vi "Update Controls in UI.vi"(4 "9216 Config":T3 {"RTD_Type" items=["TCR3851"=1, "TCR3750"=2, "TCR3916"=3, "TCR3920"=4, "TCR3911"=5, "TCR3928"=6, "Custom"=0]; "Degree Range" items=["Raw Ohms", "Degrees Kelvin", "Degrees Celsius", "Degrees Fahrenheit", "Degrees Rankine"]; "Conversion Time" items=["200 ms", "2.5 ms"]}, 6 "Values":i32[](array[numeric])=[0], 8 "RTD Type":u8, 9 "Units":u8, 10 "RTD coefficients":T1, 11 "RTD types and units controls":cluster{"controls":T2, "typedefs":T2}) -> ()   [LabVIEW 2020, in "Modules.lvlib" / "9216.lvclass"]
uses:
  9216.lvclass
  RTD Rings for Type and Units.ctl
  RTD Coefficients.ctl
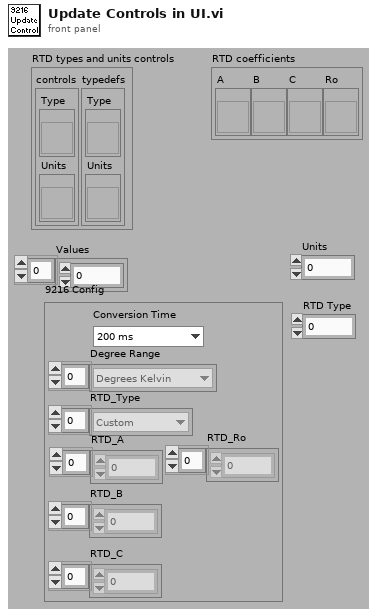
[diagram p1: front panel]
types:
  T1 = typedef "Modules.lvlib/9216.lvclass/RTD Coefficients.ctl" = cluster{"A":refnum<vi>, "B":refnum<vi>, "C":refnum<vi>, "Ro":refnum<vi>}
  T2 = typedef "Modules.lvlib/9216.lvclass/RTD Rings for Type and Units.ctl" = cluster{"Type":refnum<vi>, "Units":refnum<vi>}
  T3 = cluster{"Conversion Time":u16, "Degree Range":u8[], "RTD_Type":u8[], "RTD_A":dbl[], "RTD_B":dbl[], "RTD_C":dbl[], "RTD_Ro":dbl[]}
  T4 = typedef "LVStringsAndValuesArrayTypeDef_U8.ctl" = cluster{"String":string, "Value":u8}[]
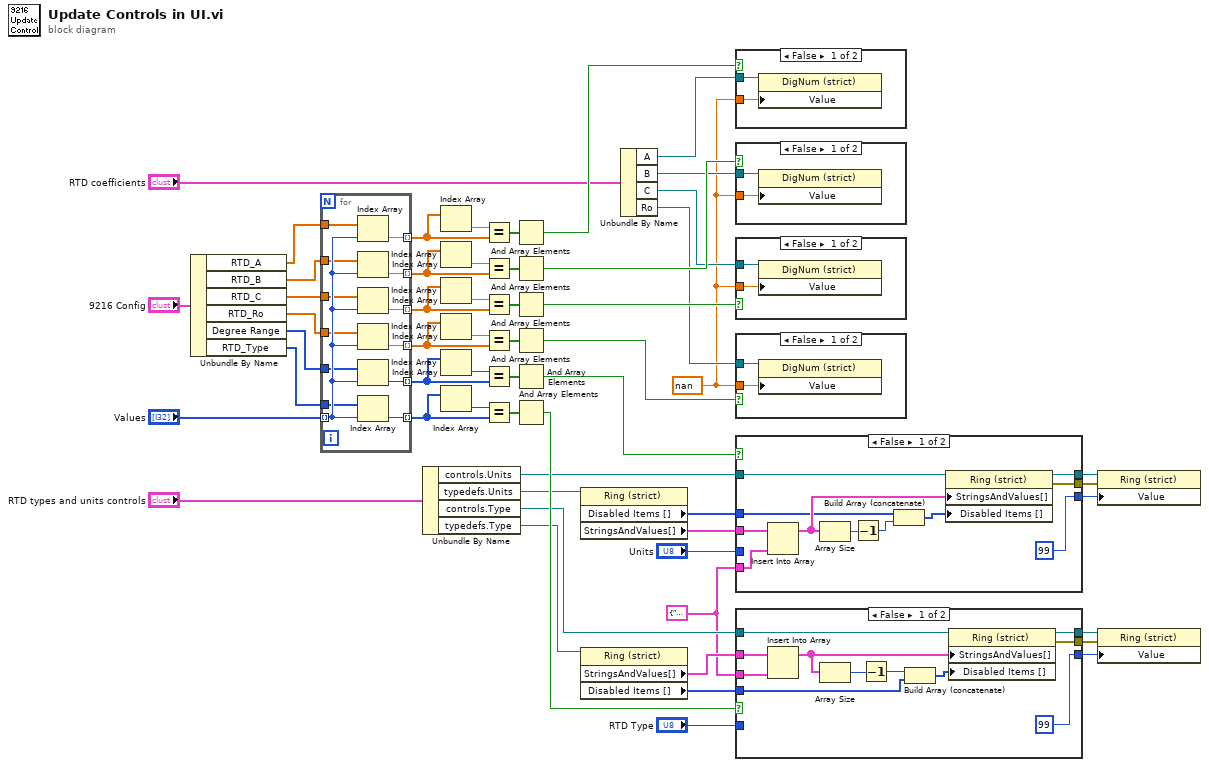
[diagram p0: block diagram]
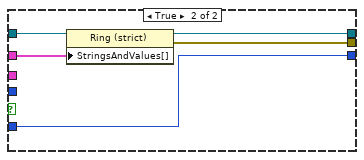
[diagram p6: hidden frame]
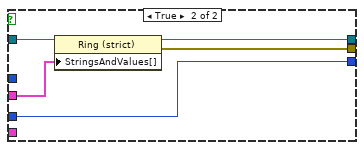
[diagram p7: hidden frame]
diagram:
  w25 = nan
  w15 = cluster{"String":string, "Value":u8} {"String"="X", "Value"=99} ("new element/subarray")
  n1 = Unbundle By Name("9216 Config") -> ("RTD_A"=w13:dbl[], "RTD_B"=w12:dbl[], "RTD_C"=w11:dbl[], "RTD_Ro"=w10:dbl[], "Degree Range"=w9:u8[], "RTD_Type"=w8:u8[])
  n2 = for {
    tunnel: "Values" -> [w67] mode=indexing
    tunnel: [w69] -> w55 mode=indexing
    tunnel: [w68] -> w54 mode=indexing
    tunnel: [w66] -> w45 mode=indexing
    tunnel: [w65] -> w46 mode=indexing
    tunnel: [w64] -> w47 mode=indexing
    tunnel: [w63] -> w48 mode=indexing
    tunnel: w9 -> [w62]
    tunnel: w8 -> [w61]
    tunnel: w13 -> [w60]
    tunnel: w12 -> [w59]
    tunnel: w11 -> [w58]
    tunnel: w10 -> [w57]
    n3 = Index Array(array=w60, index=w67) -> (element=w66:dbl)
    n4 = Index Array(array=w59, index=w67) -> (element=w65:dbl)
    n5 = Index Array(array=w58, index=w67) -> (element=w64:dbl)
    n6 = Index Array(array=w57, index=w67) -> (element=w63:dbl)
    n7 = Index Array(array=w62, index=w67) -> (element=w69:u8)
    n8 = Index Array(array=w61, index=w67) -> (element=w68:u8)
  }
  n9 = Unbundle By Name("RTD types and units controls") -> ("controls.Units"=w17:refnum<vi>, "typedefs.Units"=w16:refnum<vi>, "controls.Type"=w32:refnum<vi>, "typedefs.Type"=w31:refnum<vi>)
  n10 = Index Array(array=w45) -> (element=w21:dbl)  [unwired: 1 in]
  n11 = Index Array(array=w46) -> (element=w22:dbl)  [unwired: 1 in]
  n12 = Index Array(array=w47) -> (element=w20:dbl)  [unwired: 1 in]
  n13 = Index Array(array=w48) -> (element=w19:dbl)  [unwired: 1 in]
  n14 = Index Array(array=w55) -> (element=w24:u8)  [unwired: 1 in]
  n15 = Index Array(array=w54) -> (element=w23:u8)  [unwired: 1 in]
  n16 = Equal?(x=w21, y=w45) -> (x = y?=w41:bool[])
  n17 = Equal?(x=w22, y=w46) -> (x = y?=w42:bool[])
  n18 = Equal?(x=w20, y=w47) -> (x = y?=w43:bool[])
  n19 = Equal?(x=w19, y=w48) -> (x = y?=w44:bool[])
  n20 = Equal?(x=w24, y=w55) -> (x = y?=w53:bool[])
  n21 = Equal?(x=w23, y=w54) -> (x = y?=w52:bool[])
  n22 = And Array Elements(Boolean array=w41) -> (logical AND=w40:bool)
  n23 = And Array Elements(Boolean array=w42) -> (logical AND=w39:bool)
  n24 = And Array Elements(Boolean array=w43) -> (logical AND=w38:bool)
  n25 = And Array Elements(Boolean array=w44) -> (logical AND=w37:bool)
  n26 = And Array Elements(Boolean array=w53) -> (logical AND=w51:bool)
  n27 = And Array Elements(Boolean array=w52) -> (logical AND=w50:bool)
  n28 = property on="Property Node" class="Ring (strict)"(reference=w16) -> ("Disabled Items []"=w36:i32[], "StringsAndValues[]"=w18:T4)  [unwired: 1 in, 2 out]
  n29 = property on="Property Node" class="Ring (strict)"(reference=w31) -> ("StringsAndValues[]"=w49:T4, "Disabled Items []"=w35:i32[])  [unwired: 1 in, 2 out]
  n30 = Unbundle By Name("RTD coefficients") -> ("A"=w29:refnum<vi>, "B"=w28:refnum<vi>, "C"=w27:refnum<vi>, "Ro"=w26:refnum<vi>)
  n31 = case shown="False" w40 {
    tunnel: w29 -> [w71 _]
    tunnel: w25 -> [w70 _]
    frame False {
      n32 = property on="Property Node" class="DigNum (strict)"(reference=w71, "Value"=w70) -> ()  [unwired: 1 in, 2 out]
    }
    frame True {
    }
  }
  n33 = case shown="False" w39 {
    tunnel: w28 -> [w73 _]
    tunnel: w25 -> [w72 _]
    frame False {
      n34 = property on="Property Node" class="DigNum (strict)"(reference=w73, "Value"=w72) -> ()  [unwired: 1 in, 2 out]
    }
    frame True {
    }
  }
  n35 = case shown="False" w38 {
    tunnel: w27 -> [w75 _]
    tunnel: w25 -> [w74 _]
    frame False {
      n36 = property on="Property Node" class="DigNum (strict)"(reference=w75, "Value"=w74) -> ()  [unwired: 1 in, 2 out]
    }
    frame True {
    }
  }
  n37 = case shown="False" w37 {
    tunnel: w26 -> [w77 _]
    tunnel: w25 -> [w76 _]
    frame False {
      n38 = property on="Property Node" class="DigNum (strict)"(reference=w77, "Value"=w76) -> ()  [unwired: 1 in, 2 out]
    }
    frame True {
    }
  }
  n39 = case shown="False" w51 {
    tunnel: w18 -> [w88 w93]
    tunnel: w17 -> [w87 w92]
    tunnel: w36 -> [w80 _]
    tunnel: w15 -> [w79 _]
    tunnel: [w86 w91] -> w7
    tunnel: [w85 w90] -> w6
    tunnel: [u8 99 ("Value") w89] -> w5
    tunnel: "Units" -> [_ w89]
    frame False {
      n40 = Insert Into Array(array=w88, new element=w79) -> (w84:T4)  [unwired: 1 in]
      n41 = Array Size(array=w84) -> (size(s)=w83:i32)
      n42 = Decrement(x=w83) -> (x-1=w82:i32)
      n43 = Build Array (concatenate)(w80, w82) -> (w81:i32[])
      n44 = property on="Property Node" class="Ring (strict)"(reference=w87, "StringsAndValues[]"=w84, "Disabled Items []"=w81) -> (reference out=w86:refnum<vi>, error out=w85:errorcluster)  [unwired: 1 in]
    }
    frame True {
      n45 = property on="Property Node" class="Ring (strict)"(reference=w92, "StringsAndValues[]"=w93) -> (reference out=w91:refnum<vi>, error out=w90:errorcluster)  [unwired: 1 in]
    }
  }
  n46 = case shown="False" w50 {
    tunnel: w49 -> [w104 w109]
    tunnel: w32 -> [w103 w108]
    tunnel: w35 -> [w98 _]
    tunnel: w15 -> [w97 _]
    tunnel: "RTD Type" -> [_ w105]
    tunnel: [w96 w107] -> w3
    tunnel: [w95 w106] -> w2
    tunnel: [u8 99 ("Value") w105] -> w1
    frame False {
      n47 = Insert Into Array(array=w104, new element=w97) -> (w102:T4)  [unwired: 1 in]
      n48 = Array Size(array=w102) -> (size(s)=w101:i32)
      n49 = Decrement(x=w101) -> (x-1=w100:i32)
      n50 = Build Array (concatenate)(w100, w98) -> (w99:i32[])
      n51 = property on="Property Node" class="Ring (strict)"(reference=w103, "StringsAndValues[]"=w102, "Disabled Items []"=w99) -> (reference out=w96:refnum<vi>, error out=w95:errorcluster)  [unwired: 1 in]
    }
    frame True {
      n52 = property on="Property Node" class="Ring (strict)"(reference=w108, "StringsAndValues[]"=w109) -> (reference out=w107:refnum<vi>, error out=w106:errorcluster)  [unwired: 1 in]
    }
  }
  n53 = property on="Property Node" class="Ring (strict)"(reference=w7, error in=w6, "Value"=w5) -> ()  [unwired: 2 out]
  n54 = property on="Property Node" class="Ring (strict)"(reference=w3, error in=w2, "Value"=w1) -> ()  [unwired: 2 out]
